vi "Close.vi"(8 "Error In":errorcluster, 11 "SFTP Directory":refnum<class "SFTP Directory.lvclass">) -> (0 "Error Out":errorcluster, 3 "lv-libssh2 Shared Library":path)   [LabVIEW 2018, in "Toolkit.lvlib" / "SFTP Directory.lvclass"]
uses:
  SFTP Directory.lvclass
  SFTP Directory.lvclass/SFTP Directory.ctl
  Toolkit.lvlib
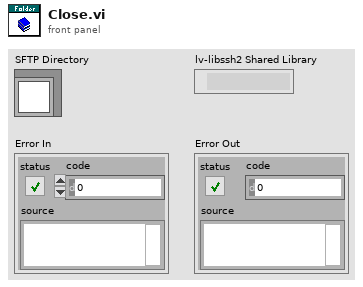
[diagram p1: front panel]
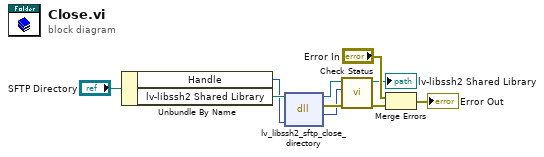
[diagram p0: block diagram]
diagram:
  n1 = Unbundle By Name("SFTP Directory") -> ("Handle"=w7:u64, "lv-libssh2 Shared Library"=w8:path)
  n2 = dll-call lib="lv-libssh2.*" fn="lv_libssh2_sftp_close_directory"(path in=w8, "handle"=w7) -> (path out=w5:path, error out=w6:errorcluster, "status"=w2:i32)  [unwired: 3 in]
  n3 = call "Check Status.vi"("Error In"=w6, "Status"=w2, "lv-libssh2 Shared Library In"=w5) -> ("Error Out"=w3:errorcluster, "lv-libssh2 Shared Library Out"=→"lv-libssh2 Shared Library":path)  [unwired: 7 in]
  n4 = Merge Errors("Error In", w3) -> (→"Error Out":errorcluster)
